vi "Calculate Phase Difference.vi"(5 "Carrier Frequency":dbl=900000000.0 format="%#_6p", 7 "Rx Device Name":refnum<k15>="192.168.10.2", 9 "Tx Device Name":refnum<k15>="192.168.10.2", 11 "error in":errorcluster) -> (6 "Phase Differences":T1, 15 "error out":errorcluster)   [LabVIEW 2015]
doc: "Calculates the phase difference between the the LO sharing channel and all other channels by injecting a common tone into all the receiving channels."
uses:
  <vilib>/measure/NI_MAPro.lvlib
  <instrlib>/niUSRP/niUSRP Timestamp.ctl
  <vilib>/measure/NI_MABase.lvlib
  <instrlib>/niUSRP/niUSRP Write Tx Data (CDB).vi
  <instrlib>/niUSRP/niUSRP Fetch Rx Data (2D CDB).vi
  <instrlib>/niUSRP/niUSRP Configure Time Start Trigger.vi
  <vilib>/Analysis/NI_AAL_Angle.lvlib
  <vilib>/Analysis/coordinate.llb/Angle Units.ctl
  <vilib>/measure/matone.llb/Extract Single Tone Information 1 Chan.vi
  <vilib>/Analysis/coordinate.llb/Wrap Angle (scalar).vi
  <vilib>/Analysis/coordinate.llb/Angle Range (Degree).ctl
  <vilib>/measure/maspectr.llb/FFT Power Spectrum for 1 Chan (CDB).vi
panel:
  in  "Start Trigger Time":T2={"whole seconds"=2, "fractional seconds"=0.0}
  out "Tx On":bool
  in  "Tone Frequency":dbl=10000.0 format="%#_6p"
  in  "Stop":bool
  in  "Rx Gain":dbl=40.0 format="%#_6f"
  in  "IQ Rate [S/sec]":dbl=1000000.0 format="%#_6p"
  out "IQ Graph":dbl[][](graph)
  out "Baseband Power Spectrum":cluster{"f0":dbl, "df":dbl, "magnitude":dbl[]}[](graph)
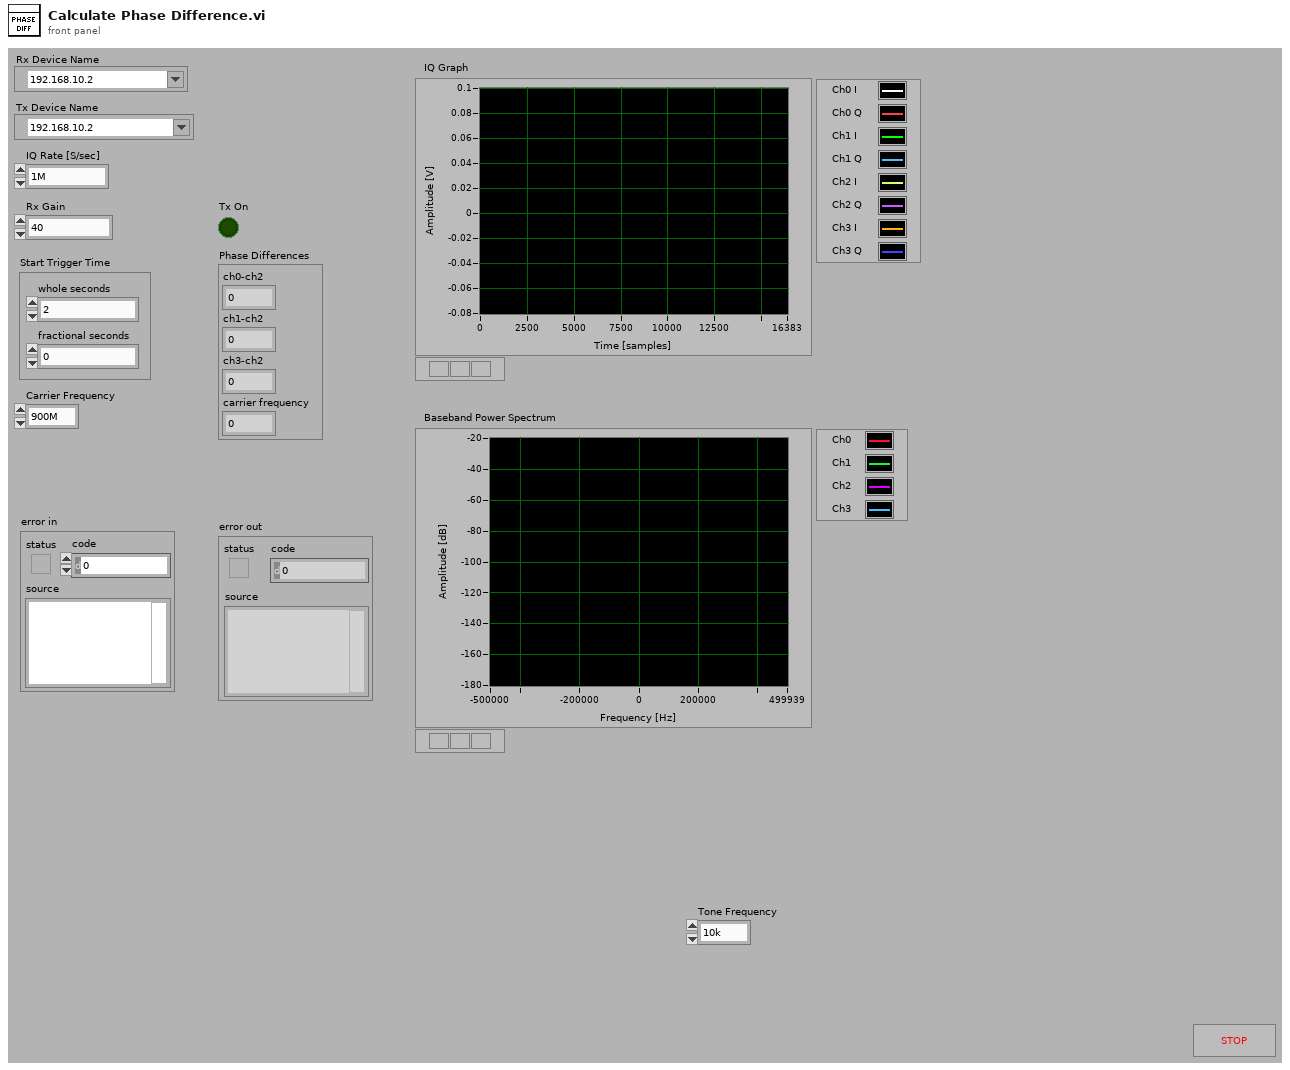
[diagram p1: front panel]
types:
  T1 = cluster{"ch0-ch2":dbl, "ch1-ch2":dbl, "ch3-ch2":dbl, "carrier frequency":dbl}
  T2 = typedef "niUSRP Timestamp.ctl" = cluster{"whole seconds":u64, "fractional seconds":dbl}
  T3 = typedef "NI_AAL_Angle.lvlib/Angle Range (Degree).ctl" = u16
  T4 = typedef "NI_AAL_Angle.lvlib/Angle Units.ctl" = i32
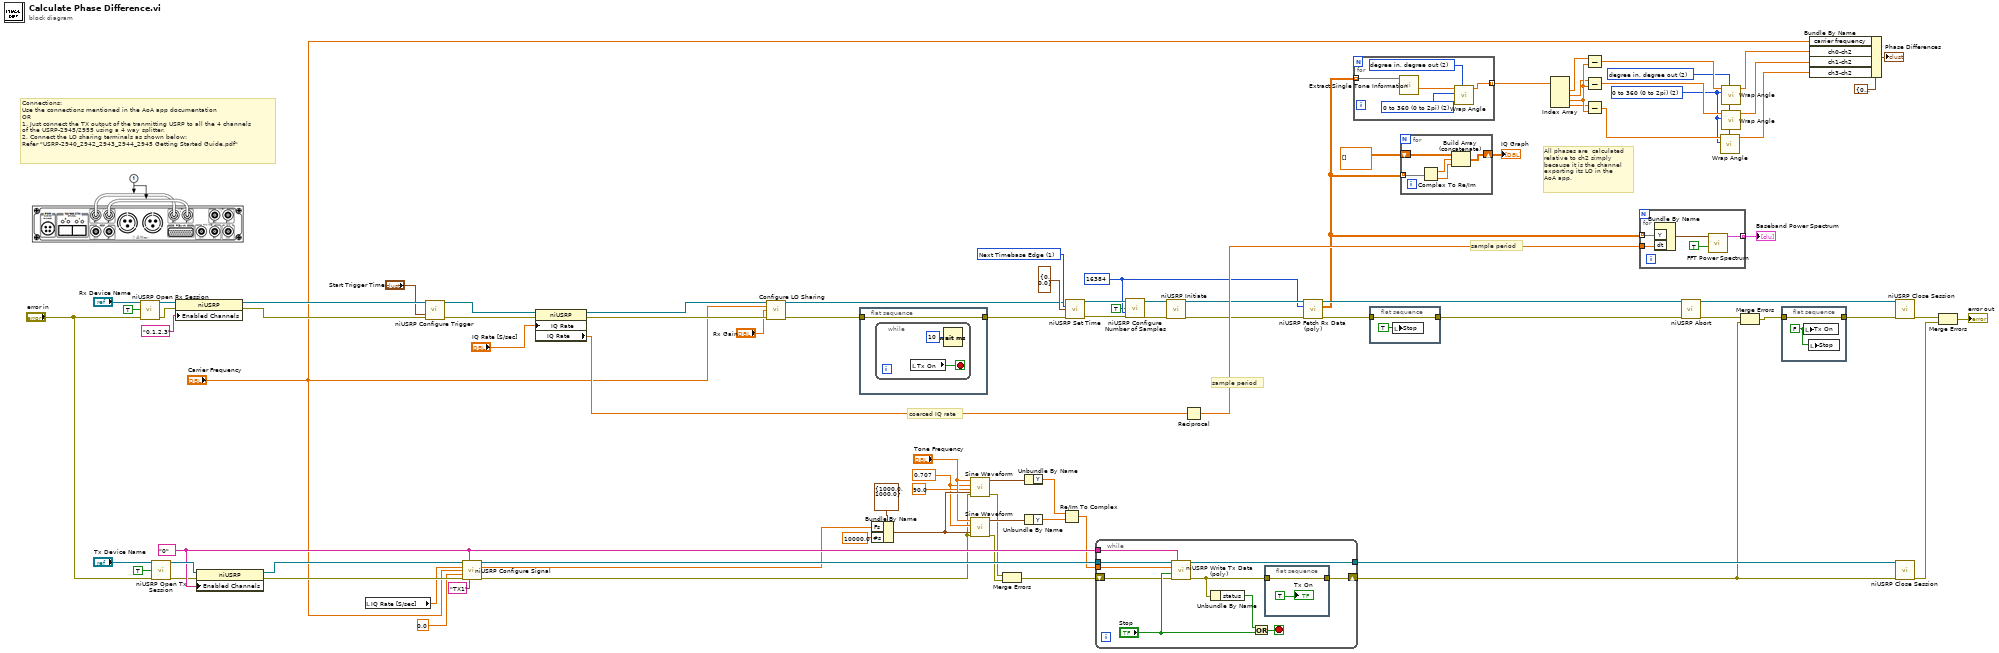
[diagram p0: block diagram]
diagram:
  w4 = T3 2 items=["none", "-180 to 180 (-pi to pi)", "0 to 360 (0 to 2pi)"] ("angle range")
  w5 = T4 2 items=["radian in, radian out", "radian in, degree out", "degree in, degree out", "degree in, radian out"] ("angle units")
  w28 = i64 16384 ("Number of Samples \nPer Fetch")
  w39 = 1 items=["Now", "Next Timebase Edge"] ("apply timestamp")
  w52 = 0.707 ("Tone Amplitude")
  w75 = "0" ("Enabled Channel")
  # "All phases are  calculated \nrelative to ch2 simply\nbecause it is the channel\nexporting its LO in the \nAoA app."
  # "sample period"
  # "sample period"
  # "coerced IQ rate"
  # "Connections:\nUse the connections mentioned in the AoA app documentation\nOR\n1. Just connect the TX output of the tranmitting USRP to all the 4 channels\nof the USRP-2945/2955 using a 4 way splitter.\n2. Connect the LO sharing terminals as shown below:\nRefer \"USRP-2940_2942_2943_2944_2945 Getting Started Guide.pdf\""
  n1 = call <instrlib>:"niUSRP Open Rx Session.vi"("device names"="Rx Device Name", "reset"=TRUE, "error in (no error)"="error in") -> ("session handle out"=w84:refnum<k15>, "error out"=w83:errorcluster)  [unwired: 11 in]
  n2 = call <instrlib>:"niUSRP Open Tx Session.vi"("device names"="Tx Device Name", "reset"=TRUE, "error in (no error)"="error in") -> ("session handle out"=w78:refnum<k15>, "error out"=w71:errorcluster)  [unwired: 11 in]
  n3 = property class="niUSRP"(reference=w84, error in=w83, "Enabled Channels"="0,1,2,3") -> (reference out=w82:refnum<k15>, error out=w81:errorcluster)
  n4 = property class="niUSRP"(reference=w78, error in=w71, "Enabled Channels"=w75) -> (reference out=w77:refnum<k15>, error out=w76:errorcluster)
  n5 = local read "IQ Rate [S/sec]"() -> (w45:dbl)
  n6 = call-poly <instrlib>:"niUSRP Configure Trigger.vi"("session handle"=w82, "start trigger time"="Start Trigger Time", "error in (no error)"=w81) -> ("session handle out"=w20:refnum<k15>, "error out"=w21:errorcluster)  [unwired: 11 in]
  n7 = call <instrlib>:"niUSRP Configure Signal.vi"("session handle"=w77, "channel list"=w75, "IQ rate"=w45, "carrier frequency"="Carrier Frequency", "gain"=0.0 ("Tx Gain"), "error in (no error)"=w76, "active antenna"="TX1" ("Tx Active Antenna")) -> ("session handle out"=w64:refnum<k15>, "coerced IQ rate"=w61:dbl, "error out"=w51:errorcluster)  [unwired: 4 in, 2 out]
  n8 = property class="niUSRP"(reference=w20, error in=w21, "IQ Rate"="IQ Rate [S/sec]") -> (reference out=w15:refnum<k15>, error out=w14:errorcluster, "IQ Rate"=w66:dbl)
  n9 = call "Configure LO Sharing.vi"("reference"=w15, "Carrier Frequency [Hz]"="Carrier Frequency", "Gain"="Rx Gain", "error in"=w14) -> ("reference out"=w13:refnum<k15>, "error out"=w12:errorcluster)  [unwired: 9 in, 1 out]
  n10 = flat-sequence {
    tunnel: [w90] -> w22
    tunnel: w12 -> [w90]
    frame #0 {
      n11 = while {
        stop <- w92 stop-if-true
        n12 = local read "Tx On"() -> (w92:bool)
        n13 = Wait (ms)(milliseconds to wait=u32 10) -> ()  [unwired: 1 out]
      }
    }
  }
  n14 = Bundle By Name(cluster=cluster{"Fs":dbl, "#s":dbl} {"Fs"=1000.0, "#s"=1000.0} ("sampling info"), "Fs"=w61, "#s"=10000.0 ("Waveform Size")) -> (w60:cluster{"Fs":dbl, "#s":dbl})
  n15 = call <vilib>:"Sine Waveform.vi"("sampling info"=w60, "error in (no error)"=w51, "phase"=90.0, "amplitude"=w52, "frequency"="Tone Frequency") -> ("error out"=w50:errorcluster, "signal out"=w57:waveform(dbl))  [unwired: 5 in]
  n16 = call <vilib>:"Sine Waveform.vi"("sampling info"=w60, "error in (no error)"=w51, "amplitude"=w52, "frequency"="Tone Frequency") -> ("error out"=w49:errorcluster, "signal out"=w58:waveform(dbl))  [unwired: 6 in]
  n17 = Merge Errors(w50, w49) -> (w48:errorcluster)
  n18 = Unbundle By Name(w57) -> ("Y"=w56:dbl[])
  n19 = Unbundle By Name(w58) -> ("Y"=w55:dbl[])
  n20 = Re/Im To Complex(1:w55, 2:w56) -> (0:w54:cdb[])
  n21 = call <instrlib>:"niUSRP Set Time.vi"("session handle"=w13, "apply timestamp"=w39, "timestamp"=T2 {"whole seconds"=0, "fractional seconds"=0.0}, "error in (no error)"=w22) -> ("session handle out"=w30:refnum<k15>, "error out"=w29:errorcluster)  [unwired: 10 in]
  n22 = while {
    tunnel: w64 -> [w96]
    tunnel: [w101] -> w80
    shift-right: [w93] -> w70
    shift-left: w48 -> [w95]
    tunnel: w54 -> [w100]
    tunnel: w75 -> [w97]
    stop <- w102 stop-if-true
    n23 = call-poly <instrlib>:"niUSRP Write Tx Data (poly).vi"("session handle"=w96, "channel list"=w97, "data"=w100, "end of data?"="Stop", "error in (no error)"=w95) -> ("session handle out"=w101:refnum<k15>, "error out"=w94:errorcluster)  [unwired: 9 in]
    n24 = Unbundle By Name(w94) -> ("status"=w99:bool)
    n25 = Or(x=w99, y="Stop") -> (x .or. y?=w102:bool)
    n26 = flat-sequence {
      tunnel: w94 -> [w104]
      tunnel: [w104] -> w93
      frame #0 {
        "Tx On" <- TRUE
      }
    }
  }
  n27 = call <instrlib>:"niUSRP Configure Number of Samples.vi"("session handle"=w30, "number of samples is finite"=TRUE, "number of samples"=w28, "error in (no error)"=w29) -> ("session handle out"=w31:refnum<k15>, "error out"=w32:errorcluster)  [unwired: 10 in]
  n28 = call <instrlib>:"niUSRP Initiate.vi"("session handle"=w31, "error in (no error)"=w32) -> ("session handle out"=w42:refnum<k15>, "error out"=w41:errorcluster)  [unwired: 12 in]
  n29 = Reciprocal(x=w66) -> (1/x=w65:dbl)
  n30 = call-poly <instrlib>:"niUSRP Fetch Rx Data (poly).vi"("session handle"=w42, "number of samples"=w28, "error in (no error)"=w41) -> ("session handle out"=w40:refnum<k15>, "data"=w34:cdb[][], "error out"=w26:errorcluster)  [unwired: 9 in, 1 out]
  n31 = for {
    tunnel: w34 -> [w109] mode=indexing
    tunnel: [w105] -> w33 mode=indexing
    w106 = T3 2 items=["none", "-180 to 180 (-pi to pi)", "0 to 360 (0 to 2pi)"] ("angle range")
    w107 = T4 2 items=["radian in, radian out", "radian in, degree out", "degree in, degree out", "degree in, radian out"] ("angle units")
    n32 = call-poly <vilib>:"Extract Single Tone Information.vi"("time signal in"=w109) -> ("detected phase (deg)"=w108:dbl)  [unwired: 5 in, 5 out]
    n33 = call-poly <vilib>:"Wrap Angle.vi"("angle units"=w107, "angle range"=w106, "angle in"=w108) -> ("angle out"=w105:dbl)  [unwired: 7 in, 1 out]
  }
  n34 = flat-sequence {
    tunnel: [w111] -> w25
    tunnel: w26 -> [w111]
    frame #0 {
      n35 = local write "Stop"(TRUE) -> ()
    }
  }
  n36 = for {
    tunnel: w34 -> [w116] mode=indexing
    shift-right: [w113] -> w35
    shift-left: dbl[][] [] -> [w112]
    n37 = Complex To Re/Im(x + iy=w116) -> (x=w115:dbl[], y=w114:dbl[])
    n38 = Build Array (concatenate)(w112, w115, w114) -> (w113:dbl[][])
  }
  "IQ Graph" <- w35
  n39 = Index Array(array=w33) -> (element #1=w18:dbl, element #2=w17:dbl, element #3=w19:dbl, element #4=w16:dbl)  [unwired: 4 in]
  n40 = Subtract(x=w18, y=w19) -> (x-y=w8:dbl)
  n41 = Subtract(x=w17, y=w19) -> (x-y=w7:dbl)
  n42 = Subtract(x=w16, y=w19) -> (x-y=w6:dbl)
  n43 = for {
    tunnel: [w121] -> w24 mode=indexing
    tunnel: w34 -> [w119] mode=indexing
    tunnel: w65 -> [w117]
    n44 = Bundle By Name("Y"=w119, "dt"=w117) -> (w118:waveform(cdb))  [unwired: 1 in]
    n45 = call-poly <vilib>:"FFT Power Spectrum.vi"("dB On (F)"=TRUE, "time signal"=w118) -> ("power spectrum"=w121:cluster{"f0":dbl, "df":dbl, "magnitude":dbl[]})  [unwired: 6 in, 3 out]
  }
  "Baseband Power Spectrum" <- w24
  n46 = call <instrlib>:"niUSRP Abort.vi"("session handle"=w40, "error in (no error)"=w25) -> ("session handle out"=w88:refnum<k15>, "error out"=w43:errorcluster)  [unwired: 12 in]
  n47 = call-poly <vilib>:"Wrap Angle.vi"("angle units"=w5, "angle range"=w4, "angle in"=w6) -> ("angle out"=w1:dbl)  [unwired: 7 in, 1 out]
  n48 = call-poly <vilib>:"Wrap Angle.vi"("angle units"=w5, "angle range"=w4, "angle in"=w8) -> ("angle out"=w3:dbl)  [unwired: 7 in, 1 out]
  n49 = call-poly <vilib>:"Wrap Angle.vi"("angle units"=w5, "angle range"=w4, "angle in"=w7) -> ("angle out"=w2:dbl)  [unwired: 7 in, 1 out]
  n50 = Merge Errors(w43, w70) -> (w44:errorcluster)
  n51 = flat-sequence {
    tunnel: w44 -> [w123]
    tunnel: [w123] -> w89
    frame #0 {
      w122 = FALSE
      n52 = local write "Tx On"(w122) -> ()
      n53 = local write "Stop"(w122) -> ()
    }
  }
  n54 = Bundle By Name(cluster=T1 {"ch0-ch2"=0.0, "ch1-ch2"=0.0, "ch3-ch2"=0.0, "carrier frequency"=0.0} ("input cluster"), "carrier frequency"="Carrier Frequency", "ch0-ch2"=w3, "ch1-ch2"=w2, "ch3-ch2"=w1) -> (→"Phase Differences":T1)
  n55 = call <instrlib>:"niUSRP Close Session.vi"("session handle"=w88, "error in (no error)"=w89) -> ("error out"=w72:errorcluster)  [unwired: 13 in]
  n56 = call <instrlib>:"niUSRP Close Session.vi"("session handle"=w80, "error in (no error)"=w70) -> ("error out"=w73:errorcluster)  [unwired: 13 in]
  n57 = Merge Errors(w72, w73) -> (→"error out":errorcluster)
